vi "M2p_AD_Std_Multi_TS.vi"() -> ()   [LabVIEW 2015]
uses:
  spcm_library/spcm_gui_m2p.llb/element_m2p_ai_channel.ctl
  spcm_library/spcm_gui_common.llb/element_mode.ctl
  spcm_library/spcm_gui_m2p.llb/element_m2p_clock.ctl
  spcm_library/spcm_gui_m2p.llb/element_m2p_ai_trigger.ctl
  spcm_library/spcm_gui_common.llb/element_device.ctl
  spcm_library/spcm_gui_common.llb/element_device_infos.ctl
  spcm_library/spcm_gui_common.llb/element_timestamps.ctl
panel:
  in  "Timestamp Settings":T1={"Mode"=2, "Timeout (RefClock)"=1000.0} {"Timeout (RefClock)" min=1.0 max=200000.0 step=1.0; "Mode" items=["Disabled", "Standard Mode", "StartReset Mode", "Standard with RefClk pos. Edge", "Standard with RefClk neg. Edge"]}
  out "Device Infos":T2={"Device Name"="M4i.4451-Exp", "Serial Number"=1122.0, "Mem (MB)"=4096.0}
  in  "Device":T3 {"Device" items=["Card", "digitizerNETBOX"]}
  in  "Trigger Settings":T4={"Trigger Source"=0, "External Trigger"=0, "Level 0 Ext"=1500, "Ext Trig Term"=FALSE, "Channel Trigger"=0, "Level 0 Ch"=0, "Level 1 Ch"=0, "Trigger Delay (Samples)"=0} {"Channel Trigger" items=["None", "Pos. Edge", "Neg. Edge", "Any Edge", "Pos. Rearm", "Neg. Rearm", "Enter Window", "Leave Window", "In Win", "Out Win"]; "External Trigger" items=["None", "Pos. Edge", "Neg. Edge", "Any Edge", "High Level", "Low Level"]; "Trigger Source" items=["Software Trigger", "External Trigger", "Channel 0 Trigger", "Channel 1 Trigger", "Channel 2 Trigger", "Channel 3 Trigger", "Channel 4 Trigger", "Channel 5 Trigger", "Channel 6 Trigger", "Channel 7 Trigger"]; "Trigger Delay (Samples)" max=65535 step=1}
  in  "Clock Settings":T5={"Clock Mode"=0, "Sampling Rate (kHz)"=10000.0, "Clock Output"=FALSE, "Termination"=FALSE, "Ref. Clock (MHz)"=10.0, "Threshold (mV)"=1500} {"Threshold (mV)" min=-5000 max=5000; "Clock Mode" items=["Internal Clock Quartz", "External Clock", "External Reference Clock"]; "Ref. Clock (MHz)" min=0.0 max=125000.0; "Sampling Rate (kHz)" min=1.0 max=5000000.0}
  in  "Mode Setup":T6={"Mode"=1, "Mem"=16384, "Seg"=4096, "Post"=2048, "Pre"=32, "ABA"=16} {"Mode" items=["Singleshot", "Multiple Recording", "Gated Sampling", "ABA Mode"]; "ABA" min=2 max=65535 step=1; "Post" min=4 step=4; "Mem" min=8 step=4; "Pre" min=4 max=8176 step=4; "Seg" min=8 step=4}
  in  "AI Channel 2":T7={"Enable"=TRUE, "Input Range "=2, "Termination"=0, "Input Type"=0, "Offset"=0} {"Input Type" items=["Single-ended", "Differential"]; "Termination" items=["1 MOhm", "50 Ohm"]; "Input Range" items=["±200 mV", "±500 mV", "±1000 mV", "±2000 mV", "±5000 mV", "±10000 mV"]}
  in  "AI Channel 7":T7={"Enable"=TRUE, "Input Range "=2, "Termination"=0, "Input Type"=0, "Offset"=0} {"Input Type" items=["Single-ended", "Differential"]; "Termination" items=["1 MOhm", "50 Ohm"]; "Input Range" items=["±200 mV", "±500 mV", "±1000 mV", "±2000 mV", "±5000 mV", "±10000 mV"]}
  in  "AI Channel 6":T7={"Enable"=TRUE, "Input Range "=2, "Termination"=0, "Input Type"=0, "Offset"=0} {"Input Type" items=["Single-ended", "Differential"]; "Termination" items=["1 MOhm", "50 Ohm"]; "Input Range" items=["±200 mV", "±500 mV", "±1000 mV", "±2000 mV", "±5000 mV", "±10000 mV"]}
  in  "AI Channel 5":T7={"Enable"=TRUE, "Input Range "=2, "Termination"=0, "Input Type"=0, "Offset"=0} {"Input Type" items=["Single-ended", "Differential"]; "Termination" items=["1 MOhm", "50 Ohm"]; "Input Range" items=["±200 mV", "±500 mV", "±1000 mV", "±2000 mV", "±5000 mV", "±10000 mV"]}
  in  "AI Channel 4":T7={"Enable"=TRUE, "Input Range "=2, "Termination"=0, "Input Type"=0, "Offset"=0} {"Input Type" items=["Single-ended", "Differential"]; "Termination" items=["1 MOhm", "50 Ohm"]; "Input Range" items=["±200 mV", "±500 mV", "±1000 mV", "±2000 mV", "±5000 mV", "±10000 mV"]}
  in  "AI Channel 3":T7={"Enable"=TRUE, "Input Range "=2, "Termination"=0, "Input Type"=0, "Offset"=0} {"Input Type" items=["Single-ended", "Differential"]; "Termination" items=["1 MOhm", "50 Ohm"]; "Input Range" items=["±200 mV", "±500 mV", "±1000 mV", "±2000 mV", "±5000 mV", "±10000 mV"]}
  in  "AI Channel 1":T7={"Enable"=TRUE, "Input Range "=2, "Termination"=0, "Input Type"=0, "Offset"=0} {"Input Type" items=["Single-ended", "Differential"]; "Termination" items=["1 MOhm", "50 Ohm"]; "Input Range" items=["±200 mV", "±500 mV", "±1000 mV", "±2000 mV", "±5000 mV", "±10000 mV"]}
  in  "AI Channel 0":T7={"Enable"=TRUE, "Input Range "=2, "Termination"=0, "Input Type"=0, "Offset"=0} {"Input Type" items=["Single-ended", "Differential"]; "Termination" items=["1 MOhm", "50 Ohm"]; "Input Range" items=["±200 mV", "±500 mV", "±1000 mV", "±2000 mV", "±5000 mV", "±10000 mV"]}
  out "Timestamps Low":u64[](array[numeric])=[2960175822456, 0, 0, 0, 0, 0, 0, 0, 0, 0, 0, 0, 0, 0, 0, 0]
  out "Timestamps High":u64[](array[numeric])
  in  "Loop Button":bool
  in  "Singleshot Button":bool=TRUE
  out "Write Setup":bool=TRUE
  out "Status":string="Acquistion finished"
  in  "Quit Button":bool
  in  "Force Trigger Button":bool
  in  "Stop Button":bool
  out "Display Data":sgl[][](graph)
  # "Range"
  # "Term"
  # "Type"
  # "Offset"
  # "Mode Settings"
  # "Ch0"
  # "Ch1"
  # "Ch2"
  # "Clock Settings"
  # "Ch3"
  # "Ch4"
  # "Ch5"
  # "Trigger Settings"
  # "Ch6"
  # "Ch7"
  # "Timestamps Settings"
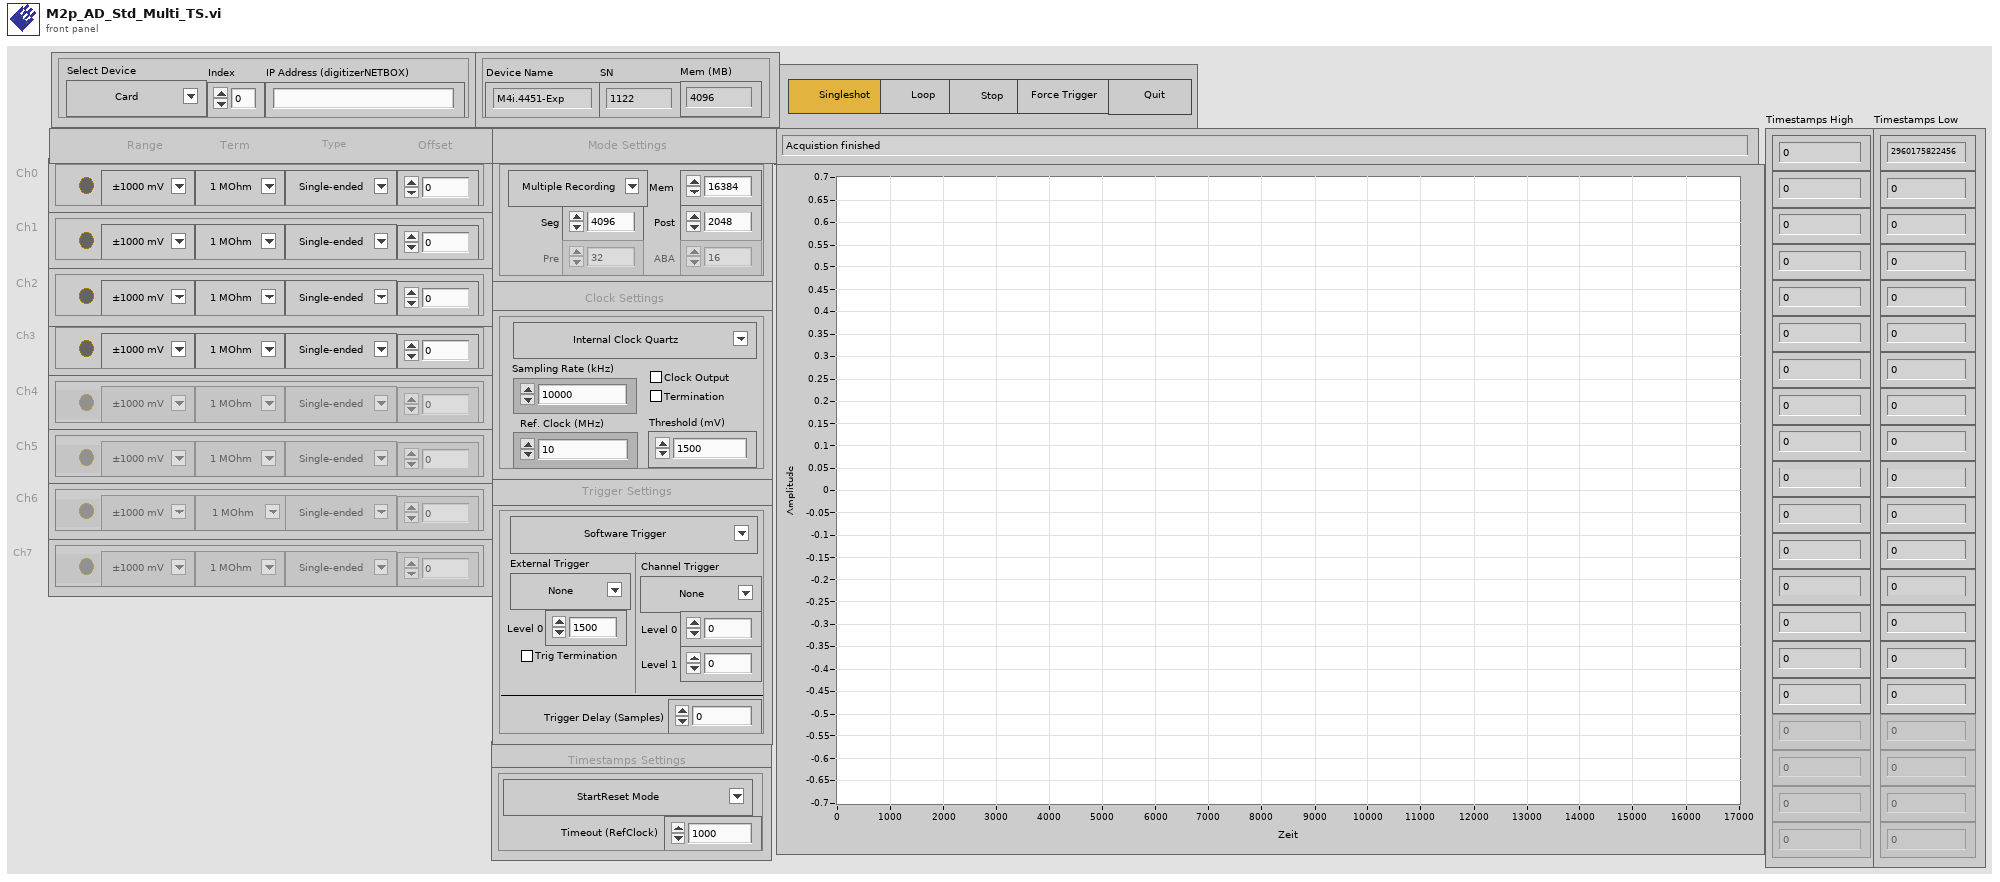
[diagram p1: front panel]
types:
  T1 = typedef "element_timestamps.ctl" = cluster{"Mode":u16, "Timeout (RefClock)":dbl}
  T2 = typedef "element_device_infos.ctl" = cluster{"Device Name":string, "Serial Number":dbl, "Mem (MB)":dbl}
  T3 = typedef "element_device.ctl" = cluster{"Index":dbl, "IP Address":string, "Device":u16}
  T4 = typedef "element_m2p_ai_trigger.ctl" = cluster{"Trigger Source":u16, "External Trigger":u16, "Level 0 Ext":i32, "Ext Trig Term":bool, "Channel Trigger":u16, "Level 0 Ch":i32, "Level 1 Ch":i32, "Trigger Delay (Samples)":u32}
  T5 = typedef "element_m2p_clock.ctl" = cluster{"Clock Mode":u16, "Sampling Rate (kHz)":dbl, "Clock Output":bool, "Termination":bool, "Ref. Clock (MHz)":dbl, "Threshold (mV)":i32}
  T6 = typedef "element_mode.ctl" = cluster{"Mode":u16, "Mem":u32, "Seg":u32, "Post":u32, "Pre":u32, "ABA":u32}
  T7 = typedef "element_m2p_ai_channel.ctl" = cluster{"Enable":bool, "Input Range ":u16, "Termination":u16, "Input Type":u16, "Offset":i32}
  T8 = enum16{"Idle", "Init", "Write Setup", "Start", "Acquire", "Read Data", "Stop", "Quit"}
  T9 = cluster{"Card Type":i32, "Inst Mem (high part)":i32, "Inst Mem (low part)":i32, "Serial Number":i32, "Function Type":i32, "Installed Features":i32, "Base Card Version":i32, "Module Version":i32, "Extension Version":i32, "Production Date":i32, "Max Sampling Rate":i32, "Max Channels":i32, "Demo Card":i32}
  T10 = cluster{"Card Name":string, "SN":i32, "Mem (MB)":i32}
  T11 = cluster{"AI Channels":i32, "AI Ranges":i32, "Input Ranges (mV)":i32[], "Programmable Offset":i32, "Termination Available":bool, "SE/Diff switchable":bool, "Offset in per cent/mV":bool, "Offset Calibration":bool, "Gain Calibration":bool, "Offset with open inputs":bool, "AI Range Strings[]":string[], "Bit Resolution":i32, "AC Coupling available":bool, "BW Limit available":bool, "AI Path count":i32}
  T12 = enum16{"Idle", "Init", "Write Setup", "Start", "Acquire", "Read Data", "Quit"}
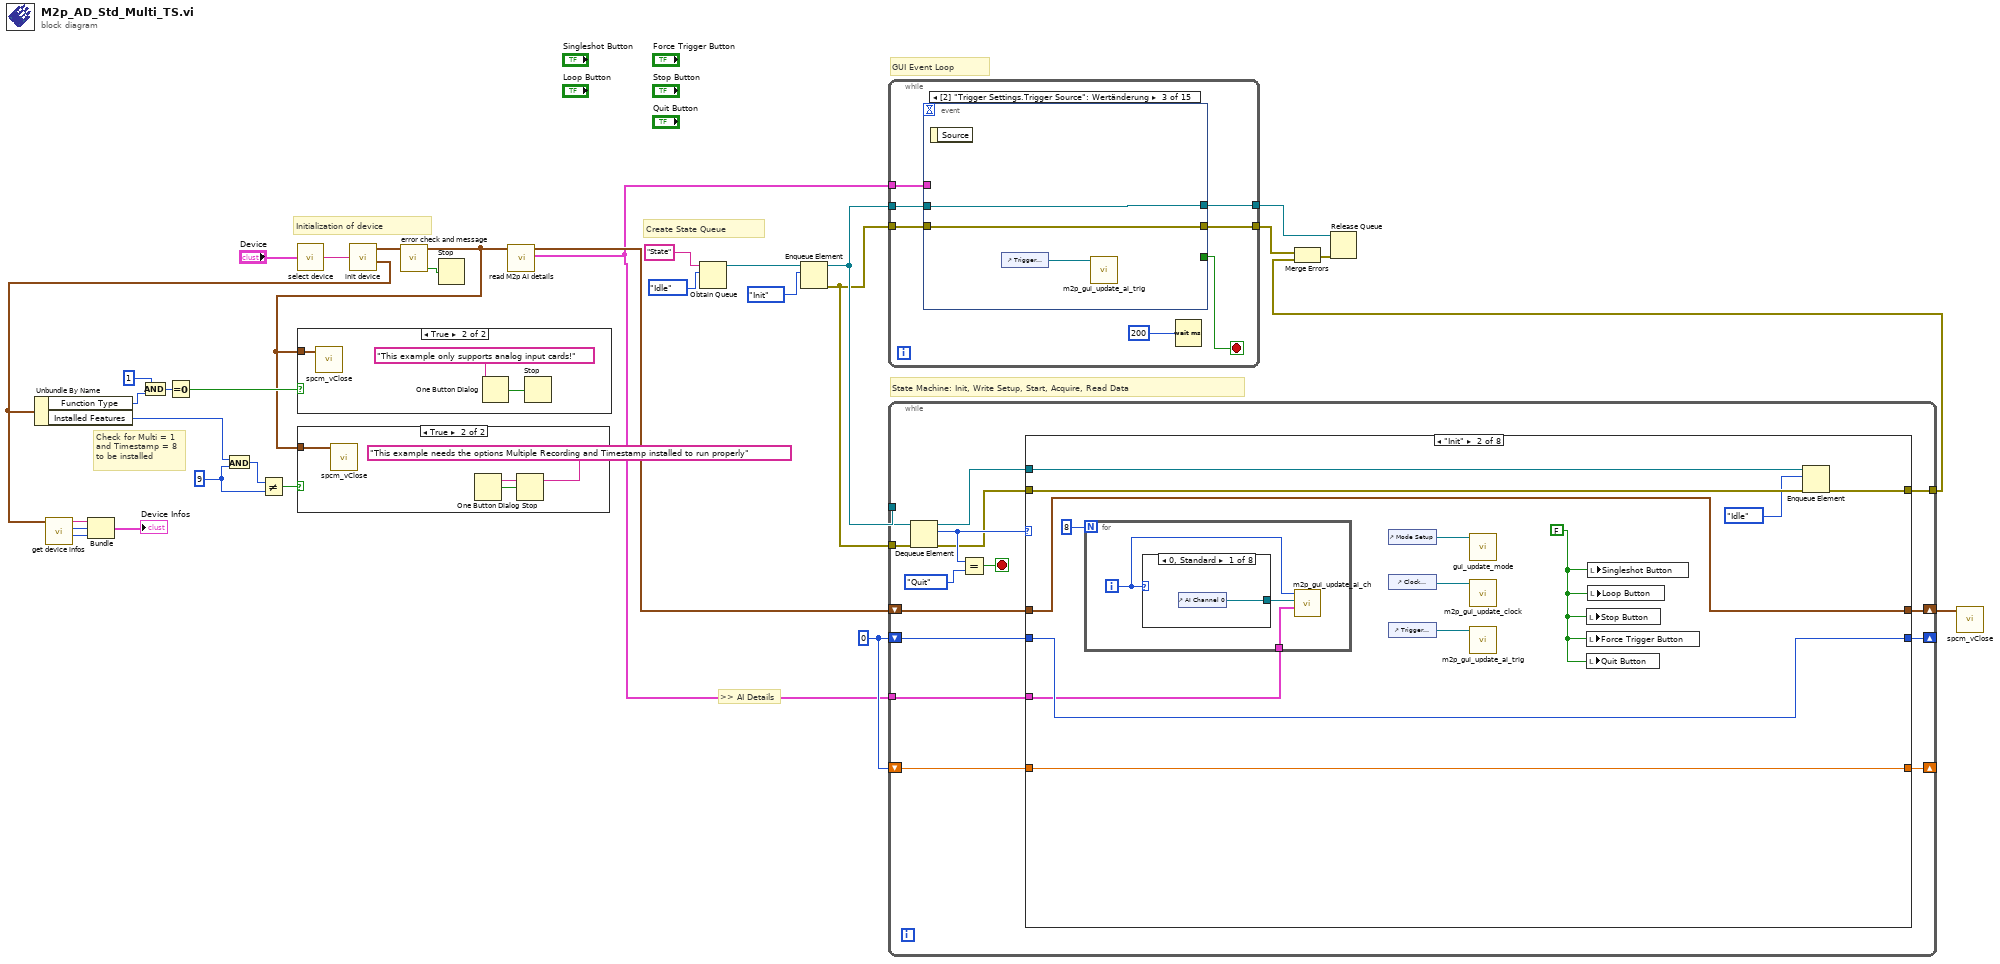
[diagram p0: block diagram]
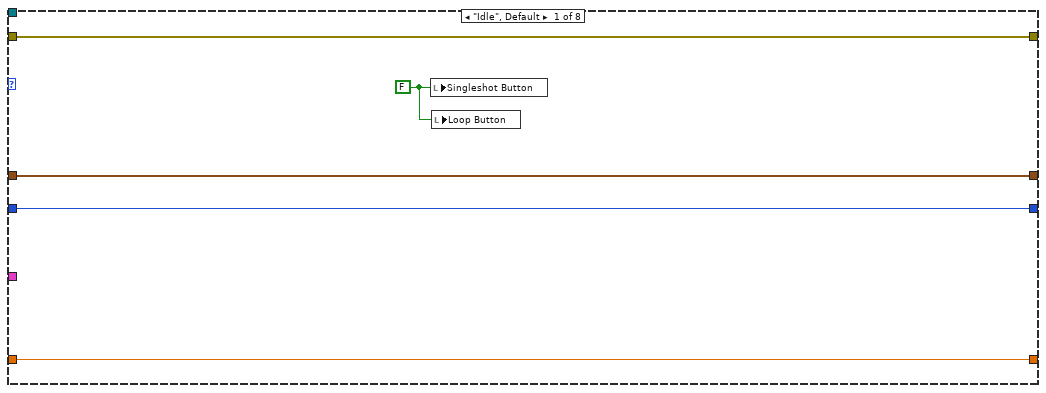
[diagram p4: hidden frame]
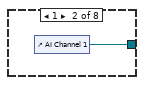
[diagram p5: hidden frame]
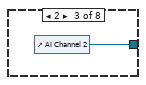
[diagram p6: hidden frame]
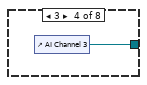
[diagram p7: hidden frame]
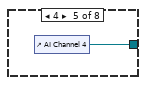
[diagram p8: hidden frame]
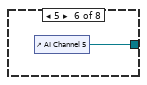
[diagram p9: hidden frame]
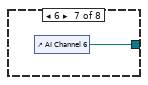
[diagram p10: hidden frame]
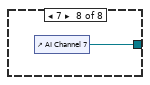
[diagram p11: hidden frame]
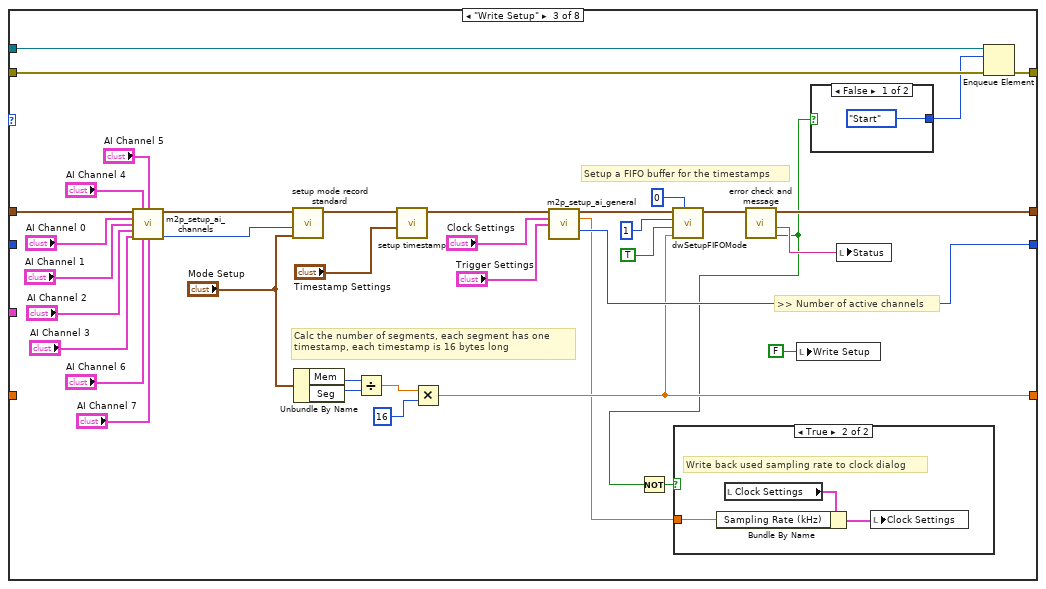
[diagram p12: hidden frame]
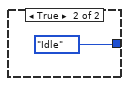
[diagram p14: hidden frame]
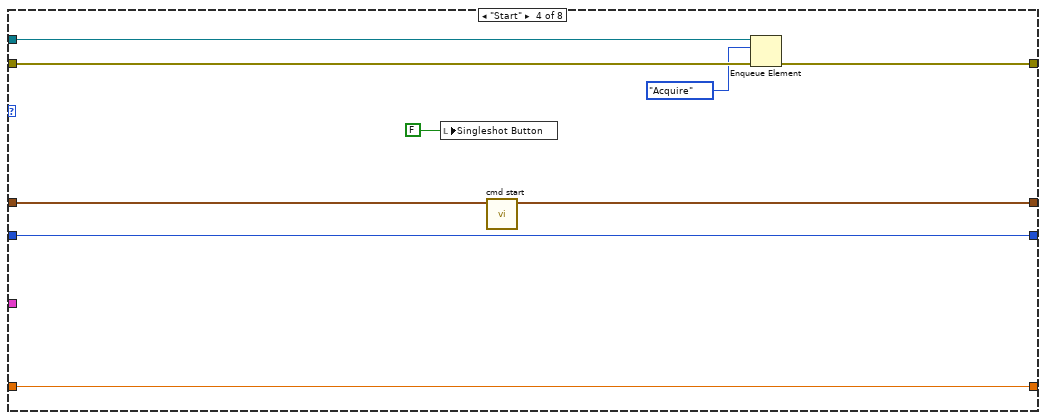
[diagram p15: hidden frame]
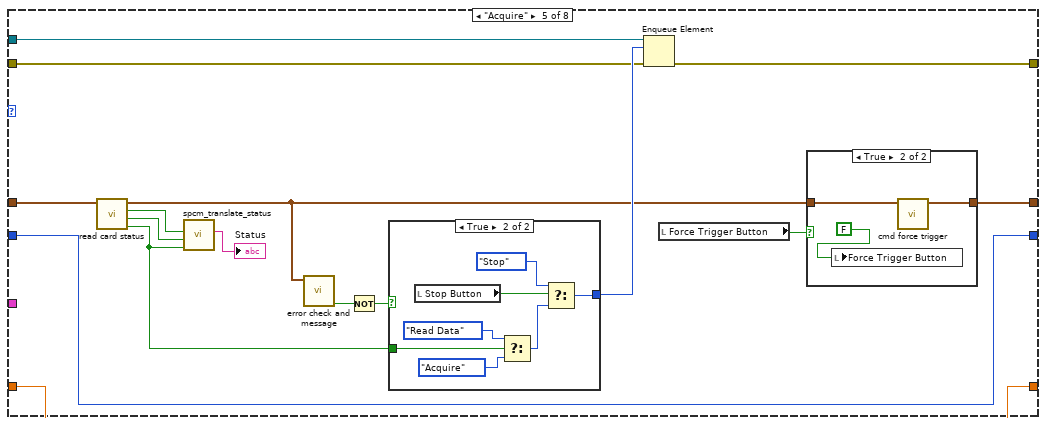
[diagram p16: hidden frame]
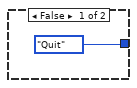
[diagram p17: hidden frame]
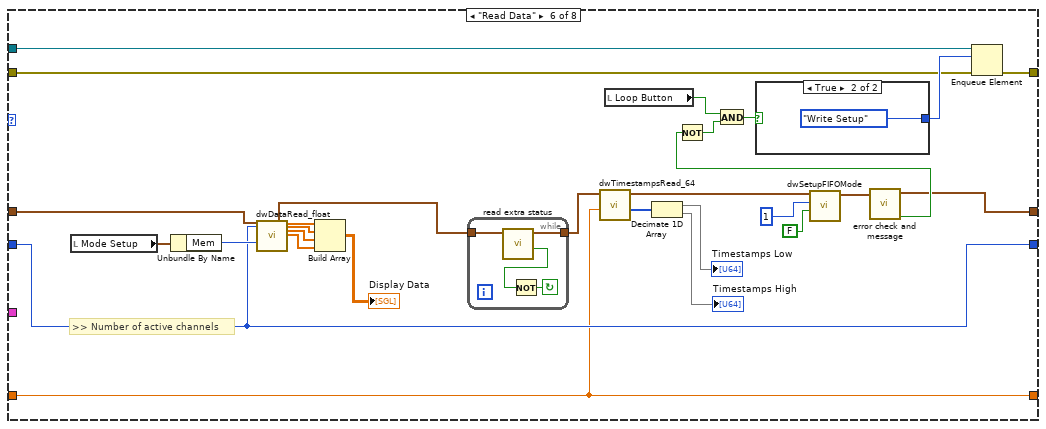
[diagram p19: hidden frame]
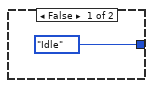
[diagram p20: hidden frame]
diagram:
  w7 = 9
  w6 = 0
  # "Check for Multi = 1\nand Timestamp = 8\nto be installed"
  # ">> AI Details"
  # "Initialization of device"
  # "Create State Queue"
  # "State Machine: Init, Write Setup, Start, Acquire, Read Data"
  # "GUI Event Loop"
  n1 = call "select device.vi"("Device"="Device") -> ("device string"=w32:string)  [unwired: 4 in]
  n2 = call "init device.vi"("Device String"=w32) -> ("Card Info Out"=w31:cluster{"Card Handle":u64, "Error Code":u32}, "Card Information"=w18:T9)  [unwired: 4 in]
  n3 = Unbundle By Name(w18) -> ("Function Type"=w22:i32, "Installed Features"=w9:i32)
  n4 = call "get device infos.vi"("Card Information"=w18) -> ("Mem (MB)"=w25:i32, "SN"=w24:i32, "Card Name"=w23:string)  [unwired: 8 in]
  n5 = Bundle("Card Name"=w23, "SN"=w24, "Mem (MB)"=w25) -> (→"Device Infos":T10)  [unwired: 1 in]
  n6 = And(x=1, y=w22) -> (x .and. y?=w21:i32)
  n7 = Equal To 0?(x=w21) -> (x = 0?=w19:bool)
  n8 = And(x=w9, y=w7) -> (x .and. y?=w8:i32)
  n9 = Not Equal?(x=w8, y=w7) -> (x != y?=w10:bool)
  n10 = call "error check and message.vi"("Card Info In"=w31) -> ("Error occurred"=w30:bool, "Card Info Out"=w5:cluster{"Card Handle":u64, "Error Code":u32})  [unwired: 4 in, 1 out]
  n11 = case shown="True" w10 {
    tunnel: w5 -> [_ w33]
    frame False {
    }
    frame True {
      n12 = call "spcm_vClose.vi"("Card Info In"=w33) -> ()  [unwired: 7 in]
      n13 = One Button Dialog(message="This example needs the options Multiple Recording and Timestamp installed to run properly") -> (true=w34:bool)  [unwired: 1 in]
      n14 = Stop(stop? (T)=w34) -> ()
    }
  }
  n15 = case shown="True" w19 {
    tunnel: w5 -> [_ w36]
    frame False {
    }
    frame True {
      n16 = call "spcm_vClose.vi"("Card Info In"=w36) -> ()  [unwired: 7 in]
      n17 = One Button Dialog(message="This example only supports analog input cards!") -> (true=w37:bool)  [unwired: 1 in]
      n18 = Stop(stop? (T)=w37) -> ()
    }
  }
  n19 = Stop(stop? (T)=w30) -> ()
  n20 = call "read M2p AI details.vi"("Card Info In"=w5) -> ("AI Details"=w3:T11, "Card Info Out"=w4:cluster{"Card Handle":u64, "Error Code":u32})  [unwired: 5 in]
  n21 = Obtain Queue(name (unnamed)="State", element data type=T8."Idle") -> (queue out=w27:refnum<queue>)  [unwired: 3 in, 2 out]
  n22 = Enqueue Element(queue=w27, element=T8."Init") -> (queue out=w28:refnum<queue>, error out=w13:errorcluster)  [unwired: 2 in, 1 out]
  n23 = while {
    tunnel: w28 -> [w43]
    tunnel: [w44] -> w14
    tunnel: [w40] -> w17
    tunnel: w13 -> [w41]
    tunnel: w3 -> [w39]
    stop <- w42 stop-if-true
    n24 = event shown="[2] \"Trigger Settings.Trigger Source\": Wertänderung" {
      selector: _ -> [_ _ _ _ _ _ _ _ _ _ _ _ _ _ _]
      dyn-events: _ -> [_ _ _ _ _ _ _ _ _ _ _ _ _ _ _]
      timeout: _ -> [_ _ _ _ _ _ _ _ _ _ _ _ _ _ _]
      tunnel: [_ _ _ _ _ _ _ _ _ _ _ _ _ TRUE _] -> w42
      tunnel: [w48 w51 w54 w59 w64 w69 w74 w79 w84 w89 w94 w99 w104 w109 w113] -> w44
      tunnel: w43 -> [w48 w51 w54 w59 w64 w69 w74 w79 w84 w89 w94 w98 w103 w110 w113]
      tunnel: [w47 w50 w53 w58 w63 w68 w73 w78 w83 w88 w93 w96 w101 w107 w112] -> w40
      tunnel: w41 -> [w47 w50 w53 w58 w63 w68 w73 w78 w83 w88 w93 w97 w102 w106 w112]
      tunnel: w39 -> [_ _ _ w57 w61 w67 w72 w77 w82 w87 w92 _ _ _ _]
      event Value Change {
        n25 = event-data ("Ereignisdatenknoten")() -> ()  [unwired: 1 in, 1 out]
        n26 = control-ref of="Mode Setup"() -> (w46:refnum<vi>)
        n27 = call "gui_update_mode.vi"("Referenz Mode Settings"=w46) -> ()  [unwired: 11 in]
      }
      event Value Change {
        n28 = event-data() -> ()  [unwired: 1 in, 1 out]
        n29 = control-ref of="Clock Settings"() -> (w49:refnum<vi>)
        n30 = call "m2p_gui_update_clock.vi"("Cluster Reference"=w49) -> ()  [unwired: 11 in]
      }
      event Value Change {
        n31 = event-data() -> ()  [unwired: 1 in, 1 out]
        n32 = control-ref of="Trigger Settings"() -> (w52:refnum<vi>)
        n33 = call "m2p_gui_update_ai_trig.vi"("Trigger Settings Reference"=w52) -> ()  [unwired: 10 in]
      }
      event Value Change {
        n34 = event-data() -> ()  [unwired: 1 in, 1 out]
        n35 = control-ref of="AI Channel 0"() -> (w56:refnum<vi>)
        n36 = call "m2p_gui_update_ai_ch.vi"("AI Details"=w57, "Cluster Referenz"=w56, "Channel Index"=0) -> ()  [unwired: 9 in]
      }
      event Value Change {
        n37 = event-data() -> ()  [unwired: 1 in, 1 out]
        n38 = control-ref of="AI Channel 1"() -> (w62:refnum<vi>)
        n39 = call "m2p_gui_update_ai_ch.vi"("AI Details"=w61, "Cluster Referenz"=w62, "Channel Index"=1) -> ()  [unwired: 9 in]
      }
      event Value Change {
        n40 = event-data() -> ()  [unwired: 1 in, 1 out]
        n41 = control-ref of="AI Channel 2"() -> (w66:refnum<vi>)
        n42 = call "m2p_gui_update_ai_ch.vi"("AI Details"=w67, "Cluster Referenz"=w66, "Channel Index"=2) -> ()  [unwired: 9 in]
      }
      event Value Change {
        n43 = event-data() -> ()  [unwired: 1 in, 1 out]
        n44 = control-ref of="AI Channel 3"() -> (w71:refnum<vi>)
        n45 = call "m2p_gui_update_ai_ch.vi"("AI Details"=w72, "Cluster Referenz"=w71, "Channel Index"=3) -> ()  [unwired: 9 in]
      }
      event Value Change {
        n46 = event-data() -> ()  [unwired: 1 in, 1 out]
        n47 = control-ref of="AI Channel 4"() -> (w75:refnum<vi>)
        n48 = call "m2p_gui_update_ai_ch.vi"("AI Details"=w77, "Cluster Referenz"=w75, "Channel Index"=4) -> ()  [unwired: 9 in]
      }
      event Value Change {
        n49 = event-data() -> ()  [unwired: 1 in, 1 out]
        n50 = control-ref of="AI Channel 5"() -> (w80:refnum<vi>)
        n51 = call "m2p_gui_update_ai_ch.vi"("AI Details"=w82, "Cluster Referenz"=w80, "Channel Index"=5) -> ()  [unwired: 9 in]
      }
      event Value Change {
        n52 = event-data() -> ()  [unwired: 1 in, 1 out]
        n53 = control-ref of="AI Channel 6"() -> (w85:refnum<vi>)
        n54 = call "m2p_gui_update_ai_ch.vi"("AI Details"=w87, "Cluster Referenz"=w85, "Channel Index"=6) -> ()  [unwired: 9 in]
      }
      event Value Change {
        n55 = event-data() -> ()  [unwired: 1 in, 1 out]
        n56 = control-ref of="AI Channel 7"() -> (w90:refnum<vi>)
        n57 = call "m2p_gui_update_ai_ch.vi"("AI Details"=w92, "Cluster Referenz"=w90, "Channel Index"=7) -> ()  [unwired: 9 in]
      }
      event "Singleshot Button", "Loop Button": Value Change {
        n58 = event-data() -> ()  [unwired: 1 in, 1 out]
        n59 = Enqueue Element(queue=w98, element=T8."Write Setup", error in (no error)=w97) -> (queue out=w99:refnum<queue>, error out=w96:errorcluster)  [unwired: 1 in, 1 out]
      }
      event "Stop Button": Value Change {
        n60 = event-data() -> ()  [unwired: 1 in, 1 out]
        n61 = Enqueue Element(queue=w103, element=T8."Idle", error in (no error)=w102) -> (queue out=w104:refnum<queue>, error out=w101:errorcluster)  [unwired: 1 in, 1 out]
      }
      event "Quit Button": Value Change {
        n62 = event-data() -> ()  [unwired: 1 in, 1 out]
        n63 = Enqueue Element(queue=w110, element=T8."Quit", error in (no error)=w106) -> (queue out=w109:refnum<queue>, error out=w107:errorcluster)  [unwired: 1 in, 1 out]
      }
      event Value Change {
        n64 = event-data() -> ()  [unwired: 1 in, 1 out]
        "Write Setup" <- TRUE
      }
    }
    n65 = Wait (ms)(milliseconds to wait=200) -> ()  [unwired: 1 out]
  }
  n66 = while {
    tunnel: w28 -> [w128]
    shift-right: [w126] -> w26
    shift-left: w4 -> [w127]
    shift-right: [w121] -> _
    shift-left: w6 -> [w122]
    tunnel: [w120] -> w16
    tunnel: w13 -> [w119]
    tunnel: w3 -> [w116]
    shift-right: [w115] -> _
    shift-left: w6 -> [w114]
    stop <- w124 stop-if-true
    n67 = Dequeue Element(queue=w128, error in (no error)=w119) -> (queue out=w123:refnum<queue>, element=w125:T8, error out=w118:errorcluster)  [unwired: 1 in, 1 out]
    n68 = Equal?(x=w125, y=T8."Quit") -> (x = y?=w124:bool)
    n69 = case shown="\"Init\"" w125 {
      tunnel: w127 -> [w133 w142 w174 w208 w215 w258 w276 w283]
      tunnel: [w133 w142 w192 w207 w222 w239 w272 w283] -> w126
      tunnel: w123 -> [_ w146 w195 w205 w219 w260 w280 _]
      tunnel: w122 -> [w132 w141 _ w209 w218 w257 w275 w282]
      tunnel: [w132 w141 w188 w209 w218 w257 w275 w282] -> w121
      tunnel: [w131 w145 w193 w204 w217 w255 w278 w284] -> w120
      tunnel: w118 -> [w131 w144 w194 w206 w216 w254 w279 w284]
      tunnel: w116 -> [_ w137 _ _ _ _ _ _]
      tunnel: [w129 w139 w176 w201 w210 w248 w273 w281] -> w115
      tunnel: w114 -> [w129 w139 _ w201 w210 w248 w273 w281]
      frame "Idle", Default {
        w130 = FALSE
        n70 = local write "Singleshot Button"(w130) -> ()
        n71 = local write "Loop Button"(w130) -> ()
      }
      frame "Init" {
        w140 = FALSE
        n72 = for {
          N: 8 -> [_]
          tunnel: w137 -> [w147]
          i -> [w148]
          n73 = case shown="0, Standard" w148 {
            tunnel: [w150 w151 w152 w153 w154 w155 w156 w157] -> w149
            frame 0, Default {
              n74 = control-ref of="AI Channel 0"() -> (w150:refnum<vi>)
            }
            frame 1 {
              n75 = control-ref of="AI Channel 1"() -> (w151:refnum<vi>)
            }
            frame 2 {
              n76 = control-ref of="AI Channel 2"() -> (w152:refnum<vi>)
            }
            frame 3 {
              n77 = control-ref of="AI Channel 3"() -> (w153:refnum<vi>)
            }
            frame 4 {
              n78 = control-ref of="AI Channel 4"() -> (w154:refnum<vi>)
            }
            frame 5 {
              n79 = control-ref of="AI Channel 5"() -> (w155:refnum<vi>)
            }
            frame 6 {
              n80 = control-ref of="AI Channel 6"() -> (w156:refnum<vi>)
            }
            frame 7 {
              n81 = control-ref of="AI Channel 7"() -> (w157:refnum<vi>)
            }
          }
          n82 = call "m2p_gui_update_ai_ch.vi"("AI Details"=w147, "Cluster Referenz"=w149, "Channel Index"=w148) -> ()  [unwired: 9 in]
        }
        n83 = control-ref of="Mode Setup"() -> (w136:refnum<vi>)
        n84 = control-ref of="Clock Settings"() -> (w135:refnum<vi>)
        n85 = control-ref of="Trigger Settings"() -> (w134:refnum<vi>)
        n86 = call "gui_update_mode.vi"("Referenz Mode Settings"=w136) -> ()  [unwired: 11 in]
        n87 = call "m2p_gui_update_clock.vi"("Cluster Reference"=w135) -> ()  [unwired: 11 in]
        n88 = call "m2p_gui_update_ai_trig.vi"("Trigger Settings Reference"=w134) -> ()  [unwired: 10 in]
        n89 = local write "Stop Button"(w140) -> ()
        n90 = local write "Force Trigger Button"(w140) -> ()
        n91 = local write "Quit Button"(w140) -> ()
        n92 = local write "Singleshot Button"(w140) -> ()
        n93 = local write "Loop Button"(w140) -> ()
        n94 = Enqueue Element(queue=w146, element=T8."Idle", error in (no error)=w144) -> (error out=w145:errorcluster)  [unwired: 1 in, 2 out]
      }
      frame "Write Setup" {
        # "Setup a FIFO buffer for the timestamps"
        # "Calc the number of segments, each segment has one\ntimestamp, each timestamp is 16 bytes long"
        # ">> Number of active channels"
        n95 = call "m2p_setup_ai_channels.vi"("Card Info In"=w174, "AI Channel 4"="AI Channel 4", "AI Channel 5"="AI Channel 5", "AI Channel 0"="AI Channel 0", "AI Channel 1"="AI Channel 1", "AI Channel 2"="AI Channel 2", "AI Channel 3"="AI Channel 3", "AI Channel 6"="AI Channel 6", "AI Channel 7"="AI Channel 7") -> ("Card Info Out"=w173:cluster{"Card Handle":u64, "Error Code":u32}, "ChMask"=w164:i32)  [unwired: 5 in]
        n96 = call "setup mode record standard.vi"("Mode Setup"="Mode Setup", "Channel Mask Low"=w164, "Card Info In"=w173) -> ("Card Info Out"=w186:cluster{"Card Handle":u64, "Error Code":u32})  [unwired: 3 in, 1 out]
        n97 = Unbundle By Name("Mode Setup") -> ("Mem"=w183:u32, "Seg"=w182:u32)
        n98 = Divide(x=w183, y=w182) -> (x/y=w181:dbl)
        n99 = call "setup timestamp.vi"("Timestamp Settings"="Timestamp Settings", "Card Info In"=w186) -> ("Card Info Out"=w184:cluster{"Card Handle":u64, "Error Code":u32})  [unwired: 4 in, 1 out]
        n100 = Multiply(x=w181, y=16) -> (x*y=w176:dbl)
        n101 = call "m2p_setup_ai_general.vi"("Card Info In"=w184, "Clock Settings"="Clock Settings", "Trigger Settings"="Trigger Settings") -> ("Card Info Out"=w185:cluster{"Card Handle":u64, "Error Code":u32}, "Used Sampling Rate (kS)"=w175:dbl, "Channel Count"=w188:i32)  [unwired: 9 in, 1 out]
        n102 = call "dwSetupFIFOMode.vi"("Notify (Bytes)"=0, "Bufferlength (Bytes)"=w176, "Allocate"=TRUE, "Buffertype (0=data, 1=TS, 2=ABA)"=1, "Card Info In"=w185) -> ("Card Info Out"=w187:cluster{"Card Handle":u64, "Error Code":u32})  [unwired: 4 in]
        n103 = call "error check and message.vi"("Card Info In"=w187) -> ("Error occurred"=w158:bool, "Error Message"=w190:string, "Card Info Out"=w192:cluster{"Card Handle":u64, "Error Code":u32})  [unwired: 4 in]
        n104 = Not(x=w158) -> (.not. x?=w159:bool)
        n105 = case shown="True" w159 {
          tunnel: w175 -> [_ w198]
          frame False {
          }
          frame True {
            # "Write back used sampling rate to clock dialog"
            n106 = local read "Clock Settings"() -> (w197:T5)
            n107 = Bundle By Name(cluster=w197, "Sampling Rate (kHz)"=w198) -> (w196:T5)
            n108 = local write "Clock Settings"(w196) -> ()
          }
        }
        n109 = local write "Write Setup"(FALSE) -> ()
        n110 = case shown="False" w158 {
          tunnel: [T8."Start" T12."Idle"] -> w191
          frame False {
          }
          frame True {
          }
        }
        n111 = local write "Status"(w190) -> ()
        n112 = Enqueue Element(queue=w195, element=w191, error in (no error)=w194) -> (error out=w193:errorcluster)  [unwired: 1 in, 2 out]
      }
      frame "Start" {
        n113 = local write "Singleshot Button"(FALSE) -> ()
        n114 = call "cmd start.vi"("Card Info In"=w208) -> ("Card Info Out"=w207:cluster{"Card Handle":u64, "Error Code":u32})  [unwired: 6 in]
        n115 = Enqueue Element(queue=w205, element=T8."Acquire", error in (no error)=w206) -> (error out=w204:errorcluster)  [unwired: 1 in, 2 out]
      }
      frame "Acquire" {
        n116 = call "read card status.vi"("Card Info In"=w215) -> ("Card ready"=w221:bool, "Trigger detected"=w224:bool, "Pretrigger full"=w225:bool, "Card Info Out"=w212:cluster{"Card Handle":u64, "Error Code":u32})  [unwired: 3 in]
        n117 = call "spcm_translate_status.vi"("Ready"=w221, "Trigger"=w224, "Pretrigger"=w225) -> ("Text"=→"Status":string)  [unwired: 4 in]
        n118 = call "error check and message.vi"("Card Info In"=w212) -> ("Error occurred"=w213:bool)  [unwired: 4 in, 2 out]
        n119 = Not(x=w213) -> (.not. x?=w214:bool)
        n120 = case shown="True" w214 {
          tunnel: [T12."Quit" w233] -> w223
          tunnel: w221 -> [_ w232]
          frame False {
          }
          frame True {
            n121 = local read "Stop Button"() -> (w227:bool)
            n122 = Select(t=T8."Read Data", s=w232, f=T8."Acquire") -> (s? t:f=w231:T8)
            n123 = Select(t=T8."Stop", s=w227, f=w231) -> (s? t:f=w233:T8)
          }
        }
        n124 = Enqueue Element(queue=w219, element=w223, error in (no error)=w216) -> (error out=w217:errorcluster)  [unwired: 1 in, 2 out]
        n125 = local read "Force Trigger Button"() -> (w211:bool)
        n126 = case shown="True" w211 {
          tunnel: w212 -> [w234 w237]
          tunnel: [w234 w236] -> w222
          frame False {
          }
          frame True {
            n127 = local write "Force Trigger Button"(FALSE) -> ()
            n128 = call "cmd force trigger.vi"("Card Info In"=w237) -> ("Card Info Out"=w236:cluster{"Card Handle":u64, "Error Code":u32})  [unwired: 6 in]
          }
        }
      }
      frame "Read Data" {
        # ">> Number of active channels"
        n129 = local read "Mode Setup"() -> (w238:T6)
        n130 = Unbundle By Name(w238) -> ("Mem"=w259:u32)
        n131 = call "dwDataRead_float.vi"("Card Info In"=w258, "Channel Count"=w257, "Length (Samples per Channel)"=w259) -> ("Card Info Out"=w250:cluster{"Card Handle":u64, "Error Code":u32}, "Ch 0"=w265:sgl[], "Ch 1"=w264:sgl[], "Ch 2"=w263:sgl[], "Ch 3"=w262:sgl[])  [unwired: 8 in, 12 out]
        n132 = Build Array(w265, w264, w263, w262) -> (→"Display Data":sgl[][])
        n133 = while {
          tunnel: w250 -> [w269]
          tunnel: [w268] -> w249
          stop <- w267 continue-if-true
          n134 = call "read extra status.vi"("Card Info In"=w269) -> ("Data transfer end"=w266:bool, "Card Info Out"=w268:cluster{"Card Handle":u64, "Error Code":u32})  [unwired: 3 in, 2 out]
          n135 = Not(x=w266) -> (.not. x?=w267:bool)
        }
        n136 = call "dwTimestampsRead_64.vi"("Length in Bytes"=w248, "Card Info In"=w249) -> ("Timestamps"=w253:u64[], "Card Info Out"=w245:cluster{"Card Handle":u64, "Error Code":u32})  [unwired: 8 in]
        n137 = local read "Loop Button"() -> (w242:bool)
        n138 = Decimate 1D Array(w253) -> (→"Timestamps Low":u64[], →"Timestamps High":u64[])
        n139 = call "dwSetupFIFOMode.vi"("Allocate"=FALSE, "Buffertype (0=data, 1=TS, 2=ABA)"=1, "Card Info In"=w245) -> ("Card Info Out"=w244:cluster{"Card Handle":u64, "Error Code":u32})  [unwired: 6 in]
        n140 = call "error check and message.vi"("Card Info In"=w244) -> ("Error occurred"=w243:bool, "Card Info Out"=w239:cluster{"Card Handle":u64, "Error Code":u32})  [unwired: 4 in, 1 out]
        n141 = Not(x=w243) -> (.not. x?=w240:bool)
        n142 = And(x=w242, y=w240) -> (x .and. y?=w241:bool)
        n143 = case shown="True" w241 {
          tunnel: [T12."Idle" T8."Write Setup"] -> w256
          frame False {
          }
          frame True {
          }
        }
        n144 = Enqueue Element(queue=w260, element=w256, error in (no error)=w254) -> (error out=w255:errorcluster)  [unwired: 1 in, 2 out]
      }
      frame "Stop" {
        n145 = call "cmd stop.vi"("Card Info In"=w276) -> ("Card Info Out"=w272:cluster{"Card Handle":u64, "Error Code":u32})  [unwired: 6 in]
        n146 = local write "Status"("Stopped") -> ()
        n147 = Enqueue Element(queue=w280, element=T8."Idle", error in (no error)=w279) -> (error out=w278:errorcluster)  [unwired: 1 in, 2 out]
      }
      frame "Quit" {
      }
    }
  }
  n148 = Merge Errors(w17, w16) -> (w15:errorcluster)
  n149 = Release Queue(queue=w14, error in (no error)=w15) -> ()  [unwired: 1 in, 3 out]
  n150 = call "spcm_vClose.vi"("Card Info In"=w26) -> ()  [unwired: 7 in]
